vi "MotorDegree.vi"(8 "Looptime":dbl, 11 "Pulse(Hz) and direction":dbl) -> (0 "MotorVel":dbl)   [LabVIEW 2019]
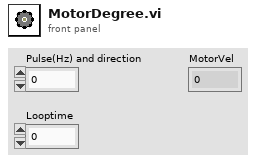
[diagram p1: front panel]
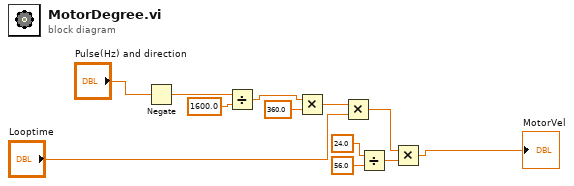
[diagram p0: block diagram]
diagram:
  n1 = Negate(x="Pulse(Hz) and direction") -> (-x=w8:dbl)
  n2 = Divide(x=w8, y=1600.0) -> (x/y=w3:dbl)
  n3 = Multiply(x=w3, y=360.0) -> (x*y=w5:dbl)
  n4 = Multiply(x=w5, y="Looptime") -> (x*y=w12:dbl)
  n5 = Divide(x=24.0, y=56.0) -> (x/y=w11:dbl)
  n6 = Multiply(x=w12, y=w11) -> (x*y=→"MotorVel":dbl)
